vi "Apply styles to GObject.vi"(8 "Error in":errorcluster, 10 "Style Sheet":T1[](array[typedef]), 11 "Gen Refnum":refnum<vi>) -> (0 "Error out":errorcluster)   [LabVIEW 2019, in "LSS.lvlib"]
doc: "This VI takes the cluster of information from a pre-parsed style sheet and applies it to a front panel element. This VI will find which class/property needs to be set, cast the front panel generic element to the right class, then apply the property desired.\n\n<b>Inputs:</b>\n<b>Gen Refnum</b> - Reference to the front panel element which will be modified.\n<b>Style Sheet</b> - Pre-parsed style sheet containing only relevent properties to apply to the control specified by Gen Refnum.\n<b>Error In</b> - Standard Error In terminal.\n\n<b>Outputs</b>\n<b>Error Out</b> - Standard Error Out terminal."
uses:
  LSS.lvlib
  Controls/Style.ctl
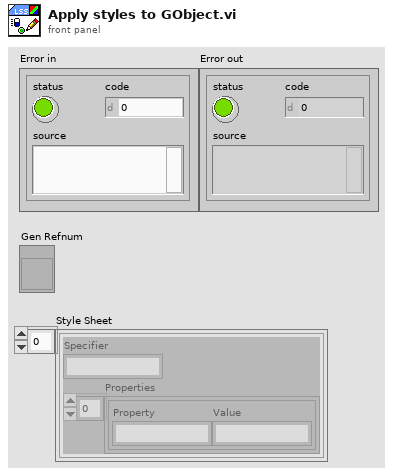
[diagram p1: front panel]
types:
  T1 = typedef "LSS.lvlib/Style.ctl" = cluster{"Specifier":string, "Properties":cluster{"Property":string, "Value":string}[]}
  T2 = enum8{"Enabled", "Disabled", "Disabled and Grayed Out"}
  T3 = enum16{"Always On", "Always Off", "Off While Running"}
  T4 = typedef "LVBoundsTypeDef.ctl" = cluster{"Width":u32, "Height":u32}
  T5 = typedef "LVRectTypeDef.ctl" = cluster{"Left":i16, "Top":i16, "Right":i16, "Bottom":i16}
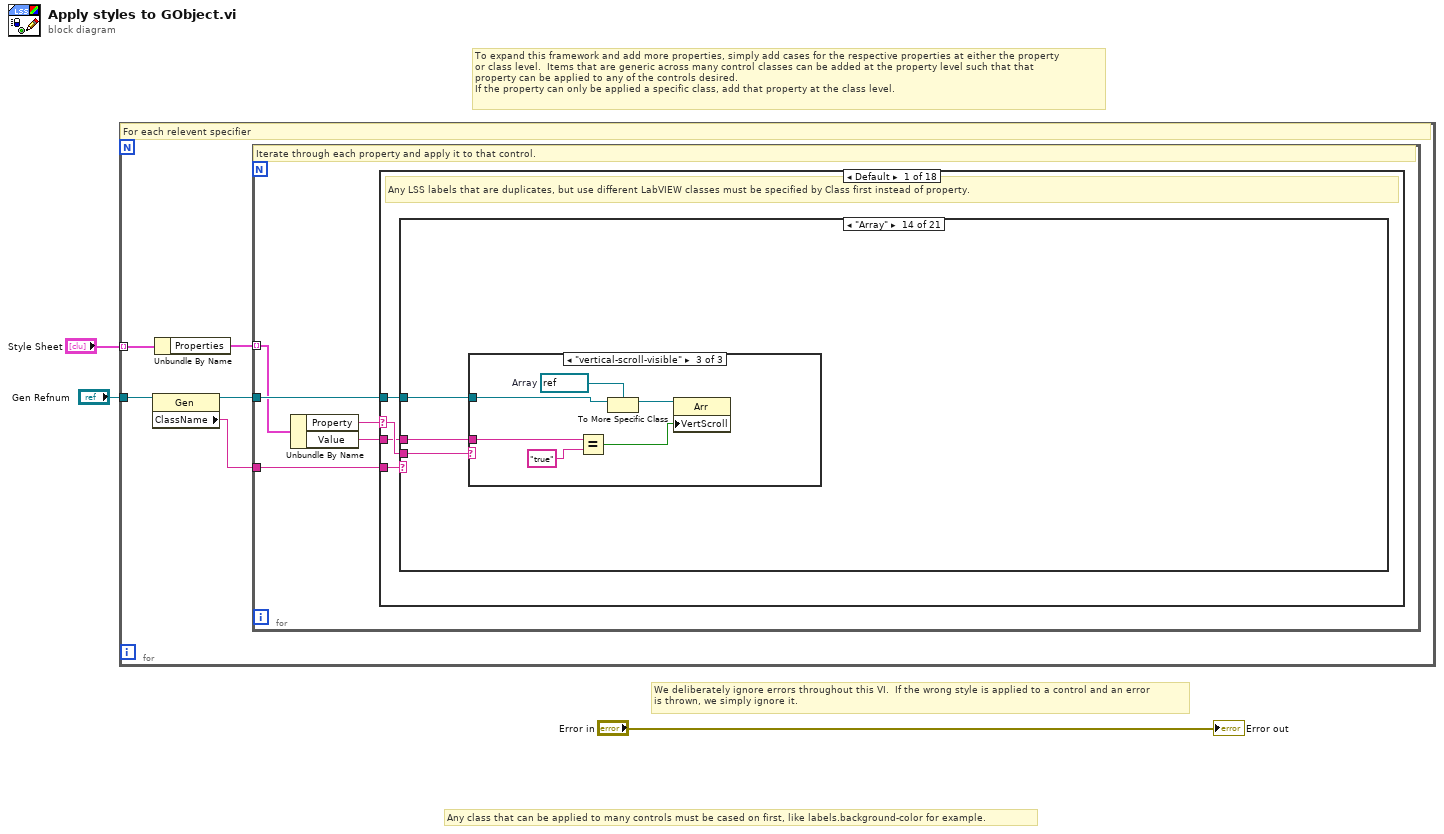
[diagram p0: block diagram]
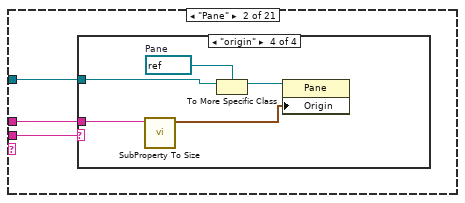
[diagram p3: hidden frame]
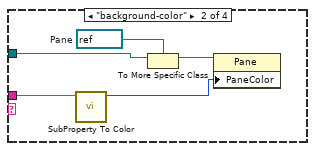
[diagram p5: hidden frame]
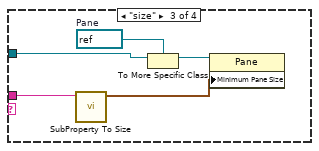
[diagram p6: hidden frame]
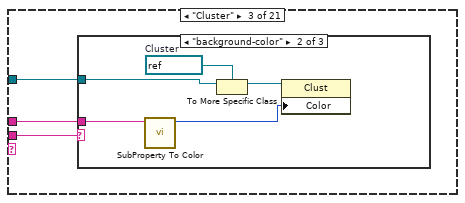
[diagram p7: hidden frame]
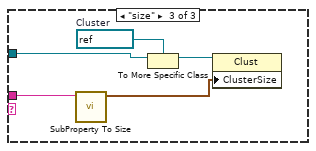
[diagram p9: hidden frame]
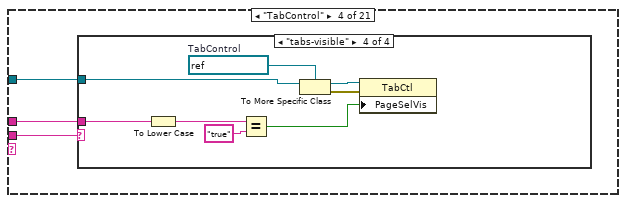
[diagram p10: hidden frame]
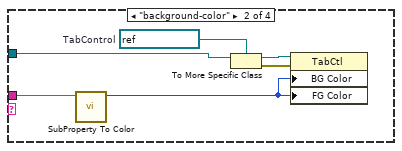
[diagram p12: hidden frame]
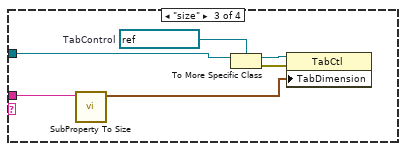
[diagram p13: hidden frame]
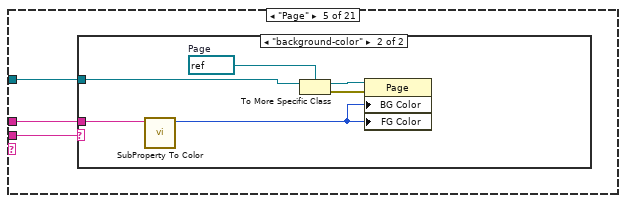
[diagram p14: hidden frame]
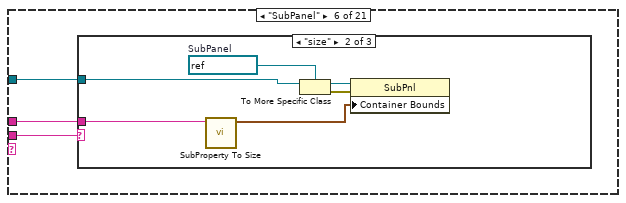
[diagram p16: hidden frame]
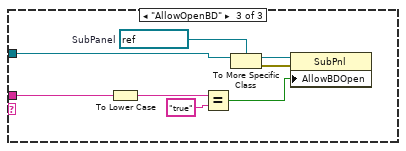
[diagram p18: hidden frame]
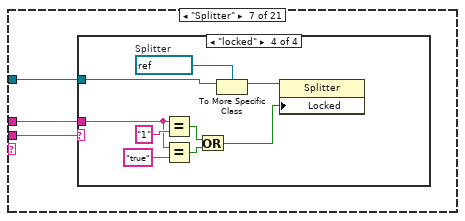
[diagram p19: hidden frame]
diagram:
  # "To expand this framework and add more properties, simply add cases for the respective properties at either the property\nor class level.  Items that are generic across many control classes can be added at the property level such that that \nproperty can be applied to any of the controls desired.\nIf the property can only be applied a specific class, add that property at the class level."
  # "Any class that can be applied to many controls must be cased on first, like labels.background-color for example."
  # "We deliberately ignore errors throughout this VI.  If the wrong style is applied to a control and an error\nis thrown, we simply ignore it."
  n1 = for {
    tunnel: "Style Sheet" -> [w8] mode=indexing
    tunnel: "Gen Refnum" -> [w6]
    # "For each relevent specifier"
    n2 = property class="Gen"(reference=w6) -> (reference out=w4:refnum<vi>, "ClassName"=w5:string)  [unwired: 1 in, 1 out]
    n3 = Unbundle By Name(w8) -> ("Properties"=w7:cluster{"Property":string, "Value":string}[])
    n4 = for {
      tunnel: w4 -> [w12]
      tunnel: w5 -> [w10]
      tunnel: w7 -> [w9] mode=indexing
      # "Iterate through each property and apply it to that control."
      n5 = Unbundle By Name(w9) -> ("Property"=w13:string, "Value"=w11:string)
      n6 = case shown="Default" w13 {
        selector: w13 -> [w16 _ _ _ _ _ _ _ _ _ _ _ _ _ _ _ _ _]
        tunnel: w12 -> [w15 w453 w458 w464 w470 w477 w483 w489 w494 w500 w507 w518 w524 w541 w555 w565 w575 w576]
        tunnel: w11 -> [w14 w449 w454 w459 w465 w473 w479 w484 w490 w495 w503 w517 w519 w530 w544 w561 w571 w579]
        tunnel: w10 -> [w17 _ _ _ _ _ _ _ _ _ _ _ _ _ _ _ _ _]
        frame Default {
          # "Any LSS labels that are duplicates, but use different LabVIEW classes must be specified by Class first instead of property."
          n7 = case shown="\"Array\"" w17 {
            selector: w17 -> [_ _ _ _ _ _ _ _ _ _ _ _ _ _ _ w255 _ _ _ _ _]
            tunnel: w16 -> [_ w20 w38 w51 w74 w83 w100 w122 w135 w153 w161 w174 w198 w220 w234 w258 w297 w324 w357 w436 w444]
            tunnel: w15 -> [_ w19 w37 w50 w73 w82 w99 w121 w134 w152 w160 w172 w197 w219 w233 w257 w296 w323 w355 w435 w443]
            tunnel: w14 -> [_ w18 w36 w49 w72 w81 w98 w120 w133 w151 w159 w173 w196 w218 w232 w256 w295 w322 w356 w432 w440]
            frame Default {
            }
            frame "Pane" {
              n8 = case shown="\"origin\"" w20 {
                tunnel: w19 -> [_ w25 w30 w35]
                tunnel: w18 -> [_ w22 w27 w32]
                frame Default {
                }
                frame "background-color" {
                  w24 = refnum<vi> refnum  # Pane
                  n9 = call "SubProperty To Color.vi"("Value"=w22) -> ("Color"=w21:u32)  [unwired: 10 in]
                  n10 = To More Specific Class(target class=w24, reference=w25) -> (specific class reference=w23:refnum<vi>)  [unwired: 1 in, 1 out]
                  n11 = property class="Pane"(reference=w23, "PaneColor"=w21) -> ()  [unwired: 1 in, 2 out]
                }
                frame "size" {
                  w29 = refnum<vi> refnum  # Pane
                  n12 = call "SubProperty To Size.vi"("SubProperty"=w27) -> ("Size"=w26:T4)  [unwired: 10 in]
                  n13 = To More Specific Class(target class=w29, reference=w30) -> (specific class reference=w28:refnum<vi>)  [unwired: 1 in, 1 out]
                  n14 = property class="Pane"(reference=w28, "Minimum Pane Size"=w26) -> ()  [unwired: 1 in, 2 out]
                }
                frame "origin" {
                  w34 = refnum<vi> refnum  # Pane
                  n15 = call "SubProperty To Size.vi"("SubProperty"=w32) -> ("Size"=w31:T4)  [unwired: 10 in]
                  n16 = To More Specific Class(target class=w34, reference=w35) -> (specific class reference=w33:refnum<vi>)  [unwired: 1 in, 1 out]
                  n17 = property class="Pane"(reference=w33, "Origin"=w31) -> ()  [unwired: 1 in, 2 out]
                }
              }
            }
            frame "Cluster" {
              n18 = case shown="\"background-color\"" w38 {
                tunnel: w37 -> [_ w43 w48]
                tunnel: w36 -> [_ w40 w45]
                frame Default {
                }
                frame "background-color" {
                  w42 = refnum<vi> refnum  # Cluster
                  n19 = call "SubProperty To Color.vi"("Value"=w40) -> ("Color"=w39:u32)  [unwired: 10 in]
                  n20 = To More Specific Class(target class=w42, reference=w43) -> (specific class reference=w41:refnum<vi>)  [unwired: 1 in, 1 out]
                  n21 = property class="Clust"(reference=w41, "Color"=w39) -> ()  [unwired: 1 in, 2 out]
                }
                frame "size" {
                  w47 = refnum<vi> refnum  # Cluster
                  n22 = call "SubProperty To Size.vi"("SubProperty"=w45) -> ("Size"=w44:T4)  [unwired: 10 in]
                  n23 = To More Specific Class(target class=w47, reference=w48) -> (specific class reference=w46:refnum<vi>)  [unwired: 1 in, 1 out]
                  n24 = property class="Clust"(reference=w46, "ClusterSize"=w44) -> ()  [unwired: 1 in, 2 out]
                }
              }
            }
            frame "TabControl" {
              n25 = case shown="\"tabs-visible\"" w51 {
                tunnel: w50 -> [_ w57 w63 w71]
                tunnel: w49 -> [_ w54 w60 w64]
                frame Default {
                }
                frame "background-color" {
                  w56 = refnum<vi> refnum  # TabControl
                  n26 = call "SubProperty To Color.vi"("Value"=w54) -> ("Color"=w52:u32)  [unwired: 10 in]
                  n27 = To More Specific Class(target class=w56, reference=w57) -> (specific class reference=w55:refnum<vi>, error out=w53:errorcluster)  [unwired: 1 in]
                  n28 = property class="TabCtl"(reference=w55, error in=w53, "BG Color"=w52, "FG Color"=w52) -> ()  [unwired: 2 out]
                }
                frame "size" {
                  w62 = refnum<vi> refnum  # TabControl
                  n29 = call "SubProperty To Size.vi"("SubProperty"=w60) -> ("Size"=w58:T4)  [unwired: 10 in]
                  n30 = To More Specific Class(target class=w62, reference=w63) -> (specific class reference=w61:refnum<vi>, error out=w59:errorcluster)  [unwired: 1 in]
                  n31 = property class="TabCtl"(reference=w61, error in=w59, "TabDimension"=w58) -> ()  [unwired: 2 out]
                }
                frame "tabs-visible" {
                  w70 = refnum<vi> refnum  # TabControl
                  n32 = To Lower Case(string=w64) -> (all lower case string=w66:string)
                  n33 = Equal?(x=w66, y="true") -> (x = y?=w65:bool)
                  n34 = To More Specific Class(target class=w70, reference=w71) -> (specific class reference=w69:refnum<vi>, error out=w68:errorcluster)  [unwired: 1 in]
                  n35 = property class="TabCtl"(reference=w69, error in=w68, "PageSelVis"=w65) -> ()  [unwired: 2 out]
                }
              }
            }
            frame "Page" {
              n36 = case shown="\"background-color\"" w74 {
                tunnel: w73 -> [_ w80]
                tunnel: w72 -> [_ w77]
                frame Default {
                }
                frame "background-color" {
                  w79 = refnum<vi> refnum  # Page
                  n37 = call "SubProperty To Color.vi"("Value"=w77) -> ("Color"=w75:u32)  [unwired: 10 in]
                  n38 = To More Specific Class(target class=w79, reference=w80) -> (specific class reference=w78:refnum<vi>, error out=w76:errorcluster)  [unwired: 1 in]
                  n39 = property class="Page"(reference=w78, error in=w76, "BG Color"=w75, "FG Color"=w75) -> ()  [unwired: 2 out]
                }
              }
            }
            frame "SubPanel" {
              n40 = case shown="\"size\"" w83 {
                tunnel: w82 -> [_ w89 w97]
                tunnel: w81 -> [_ w87 w91]
                frame Default {
                }
                frame "size" {
                  w88 = refnum<vi> refnum  # SubPanel
                  n41 = call "SubProperty To Size.vi"("SubProperty"=w87) -> ("Size"=w84:T4)  [unwired: 10 in]
                  n42 = To More Specific Class(target class=w88, reference=w89) -> (specific class reference=w86:refnum<vi>, error out=w85:errorcluster)  [unwired: 1 in]
                  n43 = property on="Property Node" class="SubPnl"(reference=w86, error in=w85, "Container Bounds"=w84) -> ()  [unwired: 2 out]
                }
                frame "AllowOpenBD" {
                  w96 = refnum<vi> refnum  # SubPanel
                  n44 = To Lower Case(string=w91) -> (all lower case string=w92:string)
                  n45 = Equal?(x=w92, y="true") -> (x = y?=w90:bool)
                  n46 = To More Specific Class(target class=w96, reference=w97) -> (specific class reference=w95:refnum<vi>, error out=w94:errorcluster)  [unwired: 1 in]
                  n47 = property on="Property Node" class="SubPnl"(reference=w95, error in=w94, "AllowBDOpen"=w90) -> ()  [unwired: 2 out]
                }
              }
            }
            frame "Splitter" {
              n48 = case shown="\"locked\"" w100 {
                tunnel: w99 -> [_ w105 w110 w119]
                tunnel: w98 -> [_ w102 w107 w113]
                frame Default {
                }
                frame "background-color" {
                  w104 = refnum<vi> refnum  # Splitter
                  n49 = call "SubProperty To Color.vi"("Value"=w102) -> ("Color"=w101:u32)  [unwired: 10 in]
                  n50 = To More Specific Class(target class=w104, reference=w105) -> (specific class reference=w103:refnum<vi>)  [unwired: 1 in, 1 out]
                  n51 = property class="Splitter"(reference=w103, "FGColor"=w101, "BGColor"=w101) -> ()  [unwired: 1 in, 2 out]
                }
                frame "splitter-position" {
                  w109 = refnum<vi> refnum  # Splitter
                  n52 = Decimal String To Number(string=w107) -> (number=w106:i32)  [unwired: 2 in, 1 out]
                  n53 = To More Specific Class(target class=w109, reference=w110) -> (specific class reference=w108:refnum<vi>)  [unwired: 1 in, 1 out]
                  n54 = property class="Splitter"(reference=w108, "Position"=w106) -> ()  [unwired: 1 in, 2 out]
                }
                frame "locked" {
                  w118 = refnum<vi> refnum  # Splitter
                  n55 = Equal?(x=w113, y="1") -> (x = y?=w116:bool)
                  n56 = Equal?(x=w113, y="true") -> (x = y?=w112:bool)
                  n57 = Or(x=w116, y=w112) -> (x .or. y?=w111:bool)
                  n58 = To More Specific Class(target class=w118, reference=w119) -> (specific class reference=w117:refnum<vi>)  [unwired: 1 in, 1 out]
                  n59 = property class="Splitter"(reference=w117, "Locked"=w111) -> ()  [unwired: 1 in, 2 out]
                }
              }
            }
            frame "RadioButtonsControl" {
              n60 = case shown="\"background-color\"" w122 {
                tunnel: w121 -> [_ w127 w132]
                tunnel: w120 -> [_ w124 w129]
                frame Default {
                }
                frame "background-color" {
                  w126 = refnum<vi> refnum  # RadioButtonsControl
                  n61 = call "SubProperty To Color.vi"("Value"=w124) -> ("Color"=w123:u32)  [unwired: 10 in]
                  n62 = To More Specific Class(target class=w126, reference=w127) -> (specific class reference=w125:refnum<vi>)  [unwired: 1 in, 1 out]
                  n63 = property class="RadioBtnsControl"(reference=w125, "Color"=w123) -> ()  [unwired: 1 in, 2 out]
                }
                frame "size" {
                  w131 = refnum<vi> refnum  # RadioButtonsControl
                  n64 = call "SubProperty To Size.vi"("SubProperty"=w129) -> ("Size"=w128:T4)  [unwired: 10 in]
                  n65 = To More Specific Class(target class=w131, reference=w132) -> (specific class reference=w130:refnum<vi>)  [unwired: 1 in, 1 out]
                  n66 = property class="RadioBtnsControl"(reference=w130, "ClusterSize"=w128) -> ()  [unwired: 1 in, 2 out]
                }
              }
            }
            frame "Decoration" {
              n67 = case shown="\"width\"" w135 {
                tunnel: w134 -> [_ w140 w145 w150]
                tunnel: w133 -> [_ w137 w142 w147]
                frame Default {
                }
                frame "background-color" {
                  w139 = refnum<vi> refnum  # Decoration
                  n68 = call "SubProperty To Color.vi"("Value"=w137) -> ("Color"=w136:u32)  [unwired: 10 in]
                  n69 = To More Specific Class(target class=w139, reference=w140) -> (specific class reference=w138:refnum<vi>)  [unwired: 1 in, 1 out]
                  n70 = property class="Decor"(reference=w138, "BG Color"=w136, "FG Color"=w136) -> ()  [unwired: 1 in, 2 out]
                }
                frame "size" {
                  w144 = refnum<vi> refnum  # Decoration
                  n71 = call "SubProperty To Size.vi"("SubProperty"=w142) -> ("Size"=w141:T4)  [unwired: 10 in]
                  n72 = To More Specific Class(target class=w144, reference=w145) -> (specific class reference=w143:refnum<vi>)  [unwired: 1 in, 1 out]
                  n73 = property class="Decor"(reference=w143, "Size"=w141) -> ()  [unwired: 1 in, 2 out]
                }
                frame "width" {
                  w149 = refnum<vi> refnum  # Decoration
                  n74 = Decimal String To Number(string=w147) -> (number=w146:i32)  [unwired: 2 in, 1 out]
                  n75 = To More Specific Class(target class=w149, reference=w150) -> (specific class reference=w148:refnum<vi>)  [unwired: 1 in, 1 out]
                  n76 = property class="Decor"(reference=w148, "Width"=w146) -> ()  [unwired: 1 in, 2 out]
                }
              }
            }
            frame "ActiveXContainer" {
              n77 = case shown="\"size\"" w153 {
                tunnel: w152 -> [_ w158]
                tunnel: w151 -> [_ w155]
                frame Default {
                }
                frame "size" {
                  w157 = refnum<vi> refnum  # ActiveXContainer
                  n78 = call "SubProperty To Size.vi"("SubProperty"=w155) -> ("Size"=w154:T4)  [unwired: 10 in]
                  n79 = To More Specific Class(target class=w157, reference=w158) -> (specific class reference=w156:refnum<vi>)  [unwired: 1 in, 1 out]
                  n80 = property class="AXCont"(reference=w156, "Container Bounds"=w154) -> ()  [unwired: 1 in, 2 out]
                }
              }
            }
            frame "Picture" {
              n81 = case shown="\"size\"" w161 {
                tunnel: w160 -> [_ w166 w171]
                tunnel: w159 -> [_ w163 w168]
                frame Default {
                }
                frame "size" {
                  w165 = refnum<vi> refnum  # Picture
                  n82 = call "SubProperty To Size.vi"("SubProperty"=w163) -> ("Size"=w162:T4)  [unwired: 10 in]
                  n83 = To More Specific Class(target class=w165, reference=w166) -> (specific class reference=w164:refnum<vi>)  [unwired: 1 in, 1 out]
                  n84 = property class="Pict"(reference=w164, "Draw Area Size"=w162) -> ()  [unwired: 1 in, 2 out]
                }
                frame "zoom" {
                  w170 = refnum<vi> refnum  # Picture
                  n85 = Fract/Exp String To Number(string=w168) -> (number=w167:dbl)  [unwired: 3 in, 1 out]
                  n86 = To More Specific Class(target class=w170, reference=w171) -> (specific class reference=w169:refnum<vi>)  [unwired: 1 in, 1 out]
                  n87 = property class="Pict"(reference=w169, "ZoomFactor"=w167) -> ()  [unwired: 1 in, 2 out]
                }
              }
            }
            frame "Boolean" {
              n88 = case shown="\"size\"" w174 {
                selector: w174 -> [w175 _ _ _ _]
                tunnel: w172 -> [_ w181 w186 w191 w195]
                tunnel: w173 -> [_ w178 w183 w188 w192]
                tunnel: [w175 _ _ _ _] -> _
                tunnel: [_ w176 _ _ _] -> _
                frame Default {
                }
                frame "size" {
                  w180 = refnum<vi> refnum  # Boolean
                  n89 = call "SubProperty To Size.vi"("SubProperty"=w178) -> ("Size"=w177:T4)  [unwired: 10 in]
                  n90 = To More Specific Class(target class=w180, reference=w181) -> (specific class reference=w179:refnum<vi>)  [unwired: 1 in, 1 out]
                  n91 = property class="Bool"(reference=w179, "Button Size"=w177) -> (error out=w176:errorcluster)  [unwired: 1 in, 1 out]
                }
                frame "font-size" {
                  w185 = refnum<vi> refnum  # Boolean
                  n92 = Decimal String To Number(string=w183) -> (number=w182:i32)  [unwired: 2 in, 1 out]
                  n93 = To More Specific Class(target class=w185, reference=w186) -> (specific class reference=w184:refnum<vi>)  [unwired: 1 in, 1 out]
                  n94 = property class="Bool"(reference=w184, "BoolText.FontSize"=w182) -> ()  [unwired: 1 in, 2 out]
                }
                frame "font-color" {
                  w190 = refnum<vi> refnum  # Boolean
                  n95 = call "SubProperty To Color.vi"("Value"=w188) -> ("Color"=w187:u32)  [unwired: 10 in]
                  n96 = To More Specific Class(target class=w190, reference=w191) -> (specific class reference=w189:refnum<vi>)  [unwired: 1 in, 1 out]
                  n97 = property class="Bool"(reference=w189, "BoolText.FontColor"=w187) -> ()  [unwired: 1 in, 2 out]
                }
                frame "font-name" {
                  w194 = refnum<vi> refnum  # Boolean
                  n98 = To More Specific Class(target class=w194, reference=w195) -> (specific class reference=w193:refnum<vi>)  [unwired: 1 in, 1 out]
                  n99 = property class="Bool"(reference=w193, "BoolText.FontName"=w192) -> ()  [unwired: 1 in, 2 out]
                }
              }
            }
            frame "Text" {
              n100 = case shown="\"background-color\"" w198 {
                tunnel: w197 -> [_ w203 w208 w213 w217]
                tunnel: w196 -> [_ w200 w205 w210 w214]
                frame Default {
                }
                frame "background-color" {
                  w202 = refnum<vi> refnum  # Text
                  n101 = call "SubProperty To Color.vi"("Value"=w200) -> ("Color"=w199:u32)  [unwired: 10 in]
                  n102 = To More Specific Class(target class=w202, reference=w203) -> (specific class reference=w201:refnum<vi>)  [unwired: 1 in, 1 out]
                  n103 = property class="Txt"(reference=w201, "BGColor"=w199, "FG Color"=w199) -> ()  [unwired: 1 in, 2 out]
                }
                frame "font-color" {
                  w207 = refnum<vi> refnum  # Text
                  n104 = call "SubProperty To Color.vi"("Value"=w205) -> ("Color"=w204:u32)  [unwired: 10 in]
                  n105 = To More Specific Class(target class=w207, reference=w208) -> (specific class reference=w206:refnum<vi>)  [unwired: 1 in, 1 out]
                  n106 = property class="Txt"(reference=w206, "TextColor"=w204) -> ()  [unwired: 1 in, 2 out]
                }
                frame "font-size" {
                  w212 = refnum<vi> refnum  # Text
                  n107 = Decimal String To Number(string=w210) -> (number=w209:i32)  [unwired: 2 in, 1 out]
                  n108 = To More Specific Class(target class=w212, reference=w213) -> (specific class reference=w211:refnum<vi>)  [unwired: 1 in, 1 out]
                  n109 = property class="Txt"(reference=w211, "FontSize"=w209) -> ()  [unwired: 1 in, 2 out]
                }
                frame "font-name" {
                  w216 = refnum<vi> refnum  # Text
                  n110 = To More Specific Class(target class=w216, reference=w217) -> (specific class reference=w215:refnum<vi>)  [unwired: 1 in, 1 out]
                  n111 = property class="Txt"(reference=w215, "FontName"=w214) -> ()  [unwired: 1 in, 2 out]
                }
              }
            }
            frame "Array" {
              n112 = case shown="\"vertical-scroll-visible\"" w220 {
                tunnel: w219 -> [_ w225 w231]
                tunnel: w218 -> [_ w222 w227]
                frame Default {
                }
                frame "numRows" {
                  w224 = refnum<vi> refnum  # Array
                  n113 = Decimal String To Number(string=w222) -> (number=w221:i32)  [unwired: 2 in, 1 out]
                  n114 = To More Specific Class(target class=w224, reference=w225) -> (specific class reference=w223:refnum<vi>)  [unwired: 1 in, 1 out]
                  n115 = property class="Arr"(reference=w223, "Number of Rows"=w221) -> ()  [unwired: 1 in, 2 out]
                }
                frame "vertical-scroll-visible" {
                  w230 = refnum<vi> refnum  # Array
                  n116 = Equal?(x=w227, y="true") -> (x = y?=w226:bool)
                  n117 = To More Specific Class(target class=w230, reference=w231) -> (specific class reference=w229:refnum<vi>)  [unwired: 1 in, 1 out]
                  n118 = property class="Arr"(reference=w229, "VertScroll"=w226) -> ()  [unwired: 1 in, 2 out]
                }
              }
            }
            frame "Enum", "Ring" {
              n119 = case shown="\"background-color\"" w234 {
                tunnel: w233 -> [_ w240 w245 w250 w254]
                tunnel: w232 -> [_ w238 w243 w248 w251]
                tunnel: [_ w235 _ _ _] -> _
                frame Default {
                }
                frame "background-color" {
                  w239 = refnum<vi> refnum  # NamedNumeric
                  n120 = call "SubProperty To Color.vi"("Value"=w238) -> ("Color"=w236:u32)  [unwired: 10 in]
                  n121 = To More Specific Class(target class=w239, reference=w240) -> (specific class reference=w237:refnum<vi>)  [unwired: 1 in, 1 out]
                  n122 = property on="Property Node" class="NmdNum"(reference=w237, "RingText.BG Color"=w236, "RingText.BGColor"=w236) -> (error out=w235:errorcluster)  [unwired: 1 in, 1 out]
                }
                frame "font-color" {
                  w241 = refnum<vi> refnum  # NamedNumeric
                  n123 = call "SubProperty To Color.vi"("Value"=w243) -> ("Color"=w242:u32)  [unwired: 10 in]
                  n124 = To More Specific Class(target class=w241, reference=w245) -> (specific class reference=w244:refnum<vi>)  [unwired: 1 in, 1 out]
                  n125 = property class="NmdNum"(reference=w244, "RingText.TextColor"=w242) -> ()  [unwired: 1 in, 2 out]
                }
                frame "font-size" {
                  w247 = refnum<vi> refnum  # NamedNumeric
                  n126 = Decimal String To Number(string=w248) -> (number=w246:i32)  [unwired: 2 in, 1 out]
                  n127 = To More Specific Class(target class=w247, reference=w250) -> (specific class reference=w249:refnum<vi>)  [unwired: 1 in, 1 out]
                  n128 = property class="NmdNum"(reference=w249, "RingText.FontSize"=w246) -> ()  [unwired: 1 in, 2 out]
                }
                frame "font-name" {
                  w252 = refnum<vi> refnum  # NamedNumeric
                  n129 = To More Specific Class(target class=w252, reference=w254) -> (specific class reference=w253:refnum<vi>)  [unwired: 1 in, 1 out]
                  n130 = property class="NmdNum"(reference=w253, "RingText.FontName"=w251) -> ()  [unwired: 1 in, 2 out]
                }
              }
            }
            frame "Knob", "Slide" {
              n131 = case shown="\"color\"" w258 {
                tunnel: w257 -> [_ w263 w266 w281 w284]
                tunnel: w256 -> [_ w260 w265 w278 w283]
                tunnel: w255 -> [_ _ w264 _ w282]
                frame Default {
                }
                frame "background-color" {
                  w262 = refnum<vi> refnum  # NumericWithScale
                  n132 = call "SubProperty To Color.vi"("Value"=w260) -> ("Color"=w259:u32)  [unwired: 10 in]
                  n133 = To More Specific Class(target class=w262, reference=w263) -> (specific class reference=w261:refnum<vi>)  [unwired: 1 in, 1 out]
                  n134 = property class="NumWthScl"(reference=w261, "BGColor"=w259, "FGColor"=w259) -> ()  [unwired: 1 in, 2 out]
                }
                frame "color" {
                  n135 = case shown="\"Slide\"" w264 {
                    tunnel: w266 -> [w271 w276]
                    tunnel: w265 -> [w268 w273]
                    frame "Slide" {
                      w270 = refnum<vi> refnum  # Slide
                      n136 = call "SubProperty To Color.vi"("Value"=w268) -> ("Color"=w267:u32)  [unwired: 10 in]
                      n137 = To More Specific Class(target class=w270, reference=w271) -> (specific class reference=w269:refnum<vi>)  [unwired: 1 in, 1 out]
                      n138 = property class="Slide"(reference=w269, "Fill Color"=w267) -> ()  [unwired: 1 in, 2 out]
                    }
                    frame "Knob", Default {
                      w275 = refnum<vi> refnum  # Knob
                      n139 = call "SubProperty To Color.vi"("Value"=w273) -> ("Color"=w272:u32)  [unwired: 10 in]
                      n140 = To More Specific Class(target class=w275, reference=w276) -> (specific class reference=w274:refnum<vi>)  [unwired: 1 in, 1 out]
                      n141 = property class="Knob"(reference=w274, "BG Color"=w272, "FG Color"=w272) -> ()  [unwired: 1 in, 2 out]
                    }
                  }
                }
                frame "size" {
                  w280 = refnum<vi> refnum  # NumericWithScale
                  n142 = call "SubProperty To Size.vi"("SubProperty"=w278) -> ("Size"=w277:T4)  [unwired: 10 in]
                  n143 = To More Specific Class(target class=w280, reference=w281) -> (specific class reference=w279:refnum<vi>)  [unwired: 1 in, 1 out]
                  n144 = property class="NumWthScl"(reference=w279, "Housing Size"=w277) -> ()  [unwired: 1 in, 2 out]
                }
                frame "font-color" {
                  n145 = case shown="\"Slide\"" w282 {
                    tunnel: w284 -> [w287 w294]
                    tunnel: w283 -> [w286 w291]
                    frame "Knob", Default {
                      w289 = refnum<vi> refnum  # Knob
                      n146 = call "SubProperty To Color.vi"("Value"=w286) -> ("Color"=w285:u32)  [unwired: 10 in]
                      n147 = To More Specific Class(target class=w289, reference=w287) -> (specific class reference=w288:refnum<vi>)  [unwired: 1 in, 1 out]
                      n148 = property class="Knob"(reference=w288, "Scale.Marker.TextColor"=w285, "Scale.MinorTickColor"=w285, "Scale.TickColor"=w285) -> ()  [unwired: 1 in, 2 out]
                    }
                    frame "Slide" {
                      w293 = refnum<vi> refnum  # Slide
                      n149 = call "SubProperty To Color.vi"("Value"=w291) -> ("Color"=w290:u32)  [unwired: 10 in]
                      n150 = To More Specific Class(target class=w293, reference=w294) -> (specific class reference=w292:refnum<vi>)  [unwired: 1 in, 1 out]
                      n151 = property class="Slide"(reference=w292, "Scale.Marker.TextColor"=w290, "Scale.MinorTickColor"=w290, "Scale.TickColor"=w290) -> ()  [unwired: 1 in, 2 out]
                    }
                  }
                }
              }
            }
            frame "String" {
              n152 = case shown="\"size\"" w297 {
                tunnel: w296 -> [_ w302 w307 w312 w317 w321]
                tunnel: w295 -> [_ w299 w304 w309 w314 w318]
                frame Default {
                }
                frame "background-color" {
                  w301 = refnum<vi> refnum  # String
                  n153 = call "SubProperty To Color.vi"("Value"=w299) -> ("Color"=w298:u32)  [unwired: 10 in]
                  n154 = To More Specific Class(target class=w301, reference=w302) -> (specific class reference=w300:refnum<vi>)  [unwired: 1 in, 1 out]
                  n155 = property class="Str"(reference=w300, "Text.BGColor"=w298) -> ()  [unwired: 1 in, 2 out]
                }
                frame "font-color" {
                  w306 = refnum<vi> refnum  # String
                  n156 = call "SubProperty To Color.vi"("Value"=w304) -> ("Color"=w303:u32)  [unwired: 10 in]
                  n157 = To More Specific Class(target class=w306, reference=w307) -> (specific class reference=w305:refnum<vi>)  [unwired: 1 in, 1 out]
                  n158 = property class="Str"(reference=w305, "Text.TextColor"=w303) -> ()  [unwired: 1 in, 2 out]
                }
                frame "size" {
                  w311 = refnum<vi> refnum  # String
                  n159 = call "SubProperty To Size.vi"("SubProperty"=w309) -> ("Size"=w308:T4)  [unwired: 10 in]
                  n160 = To More Specific Class(target class=w311, reference=w312) -> (specific class reference=w310:refnum<vi>)  [unwired: 1 in, 1 out]
                  n161 = property class="Str"(reference=w310, "Size"=w308) -> ()  [unwired: 1 in, 2 out]
                }
                frame "font-size" {
                  w316 = refnum<vi> refnum  # String
                  n162 = Decimal String To Number(string=w314) -> (number=w313:i32)  [unwired: 2 in, 1 out]
                  n163 = To More Specific Class(target class=w316, reference=w317) -> (specific class reference=w315:refnum<vi>)  [unwired: 1 in, 1 out]
                  n164 = property class="Str"(reference=w315, "Text.FontSize"=w313) -> ()  [unwired: 1 in, 2 out]
                }
                frame "font-name" {
                  w320 = refnum<vi> refnum  # String
                  n165 = To More Specific Class(target class=w320, reference=w321) -> (specific class reference=w319:refnum<vi>)  [unwired: 1 in, 1 out]
                  n166 = property class="Str"(reference=w319, "Text.FontName"=w318) -> ()  [unwired: 1 in, 2 out]
                }
              }
            }
            frame "Digital" {
              n167 = case shown="\"background-color\"" w324 {
                tunnel: w323 -> [_ w329 w334 w340 w345 w349]
                tunnel: w322 -> [_ w326 w331 w337 w342 w346]
                frame Default {
                }
                frame "background-color" {
                  w328 = refnum<vi> refnum  # Digital
                  n168 = call "SubProperty To Color.vi"("Value"=w326) -> ("Color"=w325:u32)  [unwired: 10 in]
                  n169 = To More Specific Class(target class=w328, reference=w329) -> (specific class reference=w327:refnum<vi>)  [unwired: 1 in, 1 out]
                  n170 = property class="DigNum"(reference=w327, "NumText.BG Color"=w325, "NumText.FG Color"=w325, "NumText.BGColor"=w325) -> ()  [unwired: 1 in, 2 out]
                }
                frame "font-color" {
                  w333 = refnum<vi> refnum  # Digital
                  n171 = call "SubProperty To Color.vi"("Value"=w331) -> ("Color"=w330:u32)  [unwired: 10 in]
                  n172 = To More Specific Class(target class=w333, reference=w334) -> (specific class reference=w332:refnum<vi>)  [unwired: 1 in, 1 out]
                  n173 = property class="DigNum"(reference=w332, "NumText.TextColor"=w330) -> ()  [unwired: 1 in, 2 out]
                }
                frame "size" {
                  w339 = refnum<vi> refnum  # Digital
                  n174 = call "SubProperty To Size.vi"("SubProperty"=w337) -> ("Size"=w336:T4)  [unwired: 10 in]
                  n175 = Unbundle By Name(w336) -> ("Width"=w335:u32)
                  n176 = To More Specific Class(target class=w339, reference=w340) -> (specific class reference=w338:refnum<vi>)  [unwired: 1 in, 1 out]
                  n177 = property class="DigNum"(reference=w338, "Text Width"=w335) -> ()  [unwired: 1 in, 2 out]
                }
                frame "font-size" {
                  w344 = refnum<vi> refnum  # Digital
                  n178 = Decimal String To Number(string=w342) -> (number=w341:i32)  [unwired: 2 in, 1 out]
                  n179 = To More Specific Class(target class=w344, reference=w345) -> (specific class reference=w343:refnum<vi>)  [unwired: 1 in, 1 out]
                  n180 = property class="DigNum"(reference=w343, "NumText.FontSize"=w341) -> ()  [unwired: 1 in, 2 out]
                }
                frame "font-name" {
                  w348 = refnum<vi> refnum  # Digital
                  n181 = To More Specific Class(target class=w348, reference=w349) -> (specific class reference=w347:refnum<vi>)  [unwired: 1 in, 1 out]
                  n182 = property class="DigNum"(reference=w347, "NumText.FontName"=w346) -> ()  [unwired: 1 in, 2 out]
                }
              }
            }
            frame "DigitalGraph", "GraphChart", "WaveformChart", "WaveformGraph", "XYGraph" {
              w354 = refnum<vi> refnum  # GraphChart
              n183 = To More Specific Class(target class=w354, reference=w355) -> (specific class reference=w353:refnum<vi>, error out=w350:errorcluster)  [unwired: 1 in]
              n184 = case shown="\"size\"" w357 {
                tunnel: w356 -> [_ w370 w376 w382 w388 w394 w400 w402 w407 w417 w421 w425 w431]
                tunnel: w353 -> [w364 w367 w372 w378 w384 w390 w399 w406 w411 w413 w418 w422 w427]
                tunnel: [w364 w369 w374 w380 w386 w392 w397 w404 w409 w416 w418 w422 w430] -> w352
                tunnel: [w363 w368 w373 w379 w385 w391 w395 w403 w408 w415 w419 w423 w429] -> w351
                tunnel: w350 -> [w363 w366 w375 w381 w387 w393 w398 w405 w410 w414 w420 w424 w428]
                frame Default {
                }
                frame "graph.frame-color" {
                  n185 = call "SubProperty To Color.vi"("Value"=w370) -> ("Color"=w365:u32)  [unwired: 10 in]
                  n186 = property class="GrphChrt"(reference=w367, error in=w366, "XScale.UnitLabel.BGColor"=w365, "YScale.UnitLabel.BGColor"=w365, "XScale.NameLbl.BGColor"=w365, "YScale.NameLbl.BGColor"=w365, "XScale.Marker.BGColor"=w365, "YScale.Marker.BGColor"=w365) -> ()  [unwired: 2 out]
                  n187 = property class="GrphChrt"(reference=w367, error in=w366, "Frame Color"=w365) -> (reference out=w369:refnum<vi>, error out=w368:errorcluster)
                }
                frame "graph.grid-colors.major-x" {
                  n188 = call "SubProperty To Color.vi"("Value"=w376) -> ("Color"=w371:u32)  [unwired: 10 in]
                  n189 = property class="GrphChrt"(reference=w372, error in=w375, "XScale.MajGrdColor"=w371) -> (reference out=w374:refnum<vi>, error out=w373:errorcluster)
                }
                frame "graph.grid-colors.minor-x" {
                  n190 = call "SubProperty To Color.vi"("Value"=w382) -> ("Color"=w377:u32)  [unwired: 10 in]
                  n191 = property class="GrphChrt"(reference=w378, error in=w381, "XScale.MnrGrdColor"=w377) -> (reference out=w380:refnum<vi>, error out=w379:errorcluster)
                }
                frame "graph.grid-colors.major-y" {
                  n192 = call "SubProperty To Color.vi"("Value"=w388) -> ("Color"=w383:u32)  [unwired: 10 in]
                  n193 = property class="GrphChrt"(reference=w384, error in=w387, "YScale.MajGrdColor"=w383) -> (reference out=w386:refnum<vi>, error out=w385:errorcluster)
                }
                frame "graph.grid-colors.minor-y" {
                  n194 = call "SubProperty To Color.vi"("Value"=w394) -> ("Color"=w389:u32)  [unwired: 10 in]
                  n195 = property class="GrphChrt"(reference=w390, error in=w393, "YScale.MnrGrdColor"=w389) -> (reference out=w392:refnum<vi>, error out=w391:errorcluster)
                }
                frame "font-color" {
                  n196 = call "SubProperty To Color.vi"("Value"=w400) -> ("Color"=w396:u32)  [unwired: 10 in]
                  n197 = property class="GrphChrt"(reference=w399, error in=w398, "XScale.UnitLabel.TextColor"=w396, "YScale.UnitLabel.TextColor"=w396, "XScale.NameLbl.TextColor"=w396, "YScale.NameLbl.TextColor"=w396, "XScale.Marker.TextColor"=w396, "YScale.Marker.TextColor"=w396) -> (reference out=w397:refnum<vi>, error out=w395:errorcluster)
                }
                frame "font-size" {
                  n198 = Decimal String To Number(string=w402) -> (number=w401:i32)  [unwired: 2 in, 1 out]
                  n199 = property class="GrphChrt"(reference=w406, error in=w405, "XScale.UnitLabel.FontSize"=w401, "YScale.UnitLabel.FontSize"=w401, "XScale.NameLbl.FontSize"=w401, "YScale.NameLbl.FontSize"=w401, "XScale.Marker.FontSize"=w401, "YScale.Marker.FontSize"=w401) -> (reference out=w404:refnum<vi>, error out=w403:errorcluster)
                }
                frame "font-name" {
                  n200 = property class="GrphChrt"(reference=w411, error in=w410, "XScale.UnitLabel.FontName"=w407, "YScale.UnitLabel.FontName"=w407, "XScale.NameLbl.FontName"=w407, "YScale.NameLbl.FontName"=w407, "XScale.Marker.FontName"=w407, "YScale.Marker.FontName"=w407) -> (reference out=w409:refnum<vi>, error out=w408:errorcluster)
                }
                frame "background-color" {
                  n201 = call "SubProperty To Color.vi"("Value"=w417) -> ("Color"=w412:u32)  [unwired: 10 in]
                  n202 = property class="GrphChrt"(reference=w413, error in=w414, "BG Color"=w412) -> (reference out=w416:refnum<vi>, error out=w415:errorcluster)
                }
                frame "plot-color" {
                  n203 = call "Set Plot Color.vi"("error in (no error)"=w420, "Value"=w421, "GraphChart in"=w418) -> ("error out"=w419:errorcluster)  [unwired: 8 in]
                }
                frame "line-width" {
                  n204 = call "Set Line Width.vi"("error in (no error)"=w424, "Value"=w425, "GraphChart in"=w422) -> ("error out"=w423:errorcluster)  [unwired: 8 in]
                }
                frame "size" {
                  n205 = call "SubProperty To Size.vi"("SubProperty"=w431) -> ("Size"=w426:T4)  [unwired: 10 in]
                  n206 = property class="GrphChrt"(reference=w427, error in=w428, "Plot Area Size"=w426) -> (reference out=w430:refnum<vi>, error out=w429:errorcluster)
                }
              }
              n207 = case shown="No Error" w351 {
                selector: w351 -> [w359 _]
                tunnel: w352 -> [w360 _]
                frame No Error {
                  # "Do not delete this, it refreshes the \ngraph."
                  n208 = property on="Property Node" class="GrphChrt"(reference=w360, error in=w359) -> (reference out=w361:refnum<vi>, error out=w358:errorcluster, "Plot Bounds"=w362:T5)
                  n209 = property on="Property Node" class="GrphChrt"(reference=w361, error in=w358, "Plot Bounds"=w362) -> ()  [unwired: 2 out]
                }
                frame Error {
                }
              }
            }
            frame "Table" {
              w434 = refnum<vi> refnum  # Table
              n210 = To More Specific Class(target class=w434, reference=w435) -> (specific class reference=w433:refnum<vi>)  [unwired: 1 in, 1 out]
              n211 = case shown="\"size\"" w436 {
                tunnel: w433 -> [_ w439]
                tunnel: w432 -> [_ w438]
                frame Default {
                }
                frame "size" {
                  n212 = call "SubProperty To Size.vi"("SubProperty"=w438) -> ("Size"=w437:T4)  [unwired: 10 in]
                  n213 = property class="Tbl"(reference=w439, "Size"=w437) -> ()  [unwired: 1 in, 2 out]
                }
              }
            }
            frame "Listbox" {
              w442 = refnum<vi> refnum  # ListBox
              n214 = To More Specific Class(target class=w442, reference=w443) -> (specific class reference=w441:refnum<vi>)  [unwired: 1 in, 1 out]
              n215 = case shown="\"size\"" w444 {
                tunnel: w441 -> [_ w447]
                tunnel: w440 -> [_ w446]
                frame Default {
                }
                frame "size" {
                  n216 = call "SubProperty To Size.vi"("SubProperty"=w446) -> ("Size"=w445:T4)  [unwired: 10 in]
                  n217 = property class="LstBox"(reference=w447, "Size"=w445) -> ()  [unwired: 1 in, 2 out]
                }
              }
            }
          }
        }
        frame "labels.font-size" {
          w452 = refnum<vi> refnum  # Control
          n218 = Decimal String To Number(string=w449) -> (number=w448:i32)  [unwired: 2 in, 1 out]
          n219 = To More Specific Class(target class=w452, reference=w453) -> (specific class reference=w451:refnum<vi>, error out=w450:errorcluster)  [unwired: 1 in]
          n220 = property class="Ctl"(reference=w451, error in=w450, "Label.FontSize"=w448) -> ()  [unwired: 2 out]
        }
        frame "labels.font-name" {
          w457 = refnum<vi> refnum  # Control
          n221 = To More Specific Class(target class=w457, reference=w458) -> (specific class reference=w456:refnum<vi>, error out=w455:errorcluster)  [unwired: 1 in]
          n222 = property class="Ctl"(reference=w456, error in=w455, "Label.FontName"=w454) -> ()  [unwired: 2 out]
        }
        frame "labels.font-color" {
          w463 = refnum<vi> refnum  # Control
          n223 = call "SubProperty To Color.vi"("Value"=w459) -> ("Color"=w460:u32)  [unwired: 10 in]
          n224 = To More Specific Class(target class=w463, reference=w464) -> (specific class reference=w462:refnum<vi>, error out=w461:errorcluster)  [unwired: 1 in]
          n225 = property class="Ctl"(reference=w462, error in=w461, "Label.TextColor"=w460) -> ()  [unwired: 2 out]
        }
        frame "labels.background-color" {
          w469 = refnum<vi> refnum  # Control
          n226 = call "SubProperty To Color.vi"("Value"=w465) -> ("Color"=w466:u32)  [unwired: 10 in]
          n227 = To More Specific Class(target class=w469, reference=w470) -> (specific class reference=w468:refnum<vi>, error out=w467:errorcluster)  [unwired: 1 in]
          n228 = property class="Ctl"(reference=w468, error in=w467, "Label.BGColor"=w466) -> ()  [unwired: 2 out]
        }
        frame "labels.visible" {
          w476 = refnum<vi> refnum  # Control
          n229 = Equal?(x=w473, y="true") -> (x = y?=w471:bool)
          n230 = To More Specific Class(target class=w476, reference=w477) -> (specific class reference=w475:refnum<vi>, error out=w474:errorcluster)  [unwired: 1 in]
          n231 = property class="Ctl"(reference=w475, error in=w474, "Label.Visible"=w471) -> ()  [unwired: 2 out]
        }
        frame "captions.font-size" {
          w482 = refnum<vi> refnum  # Control
          n232 = Decimal String To Number(string=w479) -> (number=w478:i32)  [unwired: 2 in, 1 out]
          n233 = To More Specific Class(target class=w482, reference=w483) -> (specific class reference=w481:refnum<vi>, error out=w480:errorcluster)  [unwired: 1 in]
          n234 = property class="Ctl"(reference=w481, error in=w480, "Caption.FontSize"=w478) -> ()  [unwired: 2 out]
        }
        frame "captions.font-color" {
          w488 = refnum<vi> refnum  # Control
          n235 = call "SubProperty To Color.vi"("Value"=w484) -> ("Color"=w485:u32)  [unwired: 10 in]
          n236 = To More Specific Class(target class=w488, reference=w489) -> (specific class reference=w487:refnum<vi>, error out=w486:errorcluster)  [unwired: 1 in]
          n237 = property class="Ctl"(reference=w487, error in=w486, "Caption.TextColor"=w485) -> ()  [unwired: 2 out]
        }
        frame "captions.font-name" {
          w493 = refnum<vi> refnum  # Control
          n238 = To More Specific Class(target class=w493, reference=w494) -> (specific class reference=w492:refnum<vi>, error out=w491:errorcluster)  [unwired: 1 in]
          n239 = property class="Ctl"(reference=w492, error in=w491, "Caption.FontName"=w490) -> ()  [unwired: 2 out]
        }
        frame "captions.background-color" {
          w499 = refnum<vi> refnum  # Control
          n240 = call "SubProperty To Color.vi"("Value"=w495) -> ("Color"=w496:u32)  [unwired: 10 in]
          n241 = To More Specific Class(target class=w499, reference=w500) -> (specific class reference=w498:refnum<vi>, error out=w497:errorcluster)  [unwired: 1 in]
          n242 = property class="Ctl"(reference=w498, error in=w497, "Caption.BGColor"=w496) -> ()  [unwired: 2 out]
        }
        frame "captions.visible" {
          w506 = refnum<vi> refnum  # Control
          n243 = Equal?(x=w503, y="true") -> (x = y?=w501:bool)
          n244 = To More Specific Class(target class=w506, reference=w507) -> (specific class reference=w505:refnum<vi>, error out=w504:errorcluster)  [unwired: 1 in]
          n245 = property class="Ctl"(reference=w505, error in=w504, "Caption.Visible"=w501) -> ()  [unwired: 2 out]
        }
        frame "position" {
          w508 = refnum<vi> refnum  # GObject
          n246 = Match Pattern(string=w517, regular expression=",") -> (before substring=w515:string, after substring=w514:string)  [unwired: 1 in, 2 out]
          n247 = call <vilib>:"Trim Whitespace.vi"("string"=w515) -> ("trimmed string"=w511:string)  [unwired: 1 in]
          n248 = call <vilib>:"Trim Whitespace.vi"("string"=w514) -> ("trimmed string"=w513:string)  [unwired: 1 in]
          n249 = To More Specific Class(target class=w508, reference=w518) -> (specific class reference=w509:refnum<vi>)  [unwired: 1 in, 1 out]
          n250 = Decimal String To Number(string=w511) -> (number=w510:i32)  [unwired: 2 in, 1 out]
          n251 = Decimal String To Number(string=w513) -> (number=w512:i32)  [unwired: 2 in, 1 out]
          n252 = property class="GObj"(reference=w509, "Left"=w510, "Top"=w512) -> ()  [unwired: 1 in, 2 out]
        }
        frame "disabled-state" {
          w523 = refnum<vi> refnum  # Control
          n253 = case shown="\"disabled\", \"true\", Default" w519 {
            tunnel: [T2."Disabled" ("Disabled") T2."Disabled and Grayed Out" ("Disabled") T2."Enabled" ("Disabled")] -> w520
            frame "disabled", "true", Default {
            }
            frame "gray" {
            }
            frame "enabled", "false" {
            }
          }
          n254 = To More Specific Class(target class=w523, reference=w524) -> (specific class reference=w522:refnum<vi>, error out=w521:errorcluster)  [unwired: 1 in]
          n255 = property class="Ctl"(reference=w522, error in=w521, "DisabledEnum"=w520) -> ()  [unwired: 2 out]
        }
        frame "bool.true-color" {
          w540 = refnum<vi> refnum  # Boolean
          n256 = call "SubProperty To Color.vi"("Value"=w530) -> ("Color"=w534:u32)  [unwired: 10 in]
          n257 = To More Specific Class(target class=w540, reference=w541) -> (specific class reference=w538:refnum<vi>, error out=w539:errorcluster)  [unwired: 1 in]
          n258 = Bundle(cluster=cluster{u32, u32} {0, 0}, w534, w534) -> (w528:cluster{u32, u32})
          n259 = property class="Bool"(reference=w538, error in=w539) -> (reference out=w536:refnum<vi>, error out=w537:errorcluster, "Colors [4]"=w535:cluster{u32, u32}[])
          n260 = Replace Array Subset(array=w535, new element #1=w528, index #1=1 ("index"), new element #2=w528, index #2=3 ("index")) -> (w531:cluster{u32, u32}[])
          n261 = property class="Bool"(reference=w536, error in=w537, "Colors [4]"=w531) -> ()  [unwired: 2 out]
        }
        frame "bool.false-color" {
          w554 = refnum<vi> refnum  # Boolean
          n262 = call "SubProperty To Color.vi"("Value"=w544) -> ("Color"=w548:u32)  [unwired: 10 in]
          n263 = To More Specific Class(target class=w554, reference=w555) -> (specific class reference=w552:refnum<vi>, error out=w553:errorcluster)  [unwired: 1 in]
          n264 = Bundle(cluster=cluster{u32, u32} {0, 0}, w548, w548) -> (w542:cluster{u32, u32})
          n265 = property class="Bool"(reference=w552, error in=w553) -> (reference out=w550:refnum<vi>, error out=w551:errorcluster, "Colors [4]"=w549:cluster{u32, u32}[])
          n266 = Replace Array Subset(array=w549, new element #1=w542, index #1=0 ("index"), new element #2=w542, index #2=2 ("index")) -> (w545:cluster{u32, u32}[])
          n267 = property class="Bool"(reference=w550, error in=w551, "Colors [4]"=w545) -> ()  [unwired: 2 out]
        }
        frame "horizontal-scroll-bar" {
          w564 = refnum<vi> refnum  # Pane
          n268 = Equal?(x=w561, y="true") -> (x = y?=w559:bool)
          n269 = Select(t=T3."Always On" ("Horizontal Scrollbar Visibility"), s=w559, f=T3."Always Off" ("Horizontal Scrollbar Visibility")) -> (s? t:f=w556:T3)
          n270 = To More Specific Class(target class=w564, reference=w565) -> (specific class reference=w563:refnum<vi>, error out=w562:errorcluster)  [unwired: 1 in]
          n271 = property class="Pane"(reference=w563, error in=w562, "HorizScrollbarVisibility"=w556) -> ()  [unwired: 2 out]
        }
        frame "vertical-scroll-bar" {
          w574 = refnum<vi> refnum  # Pane
          n272 = Equal?(x=w571, y="true") -> (x = y?=w569:bool)
          n273 = Select(t=T3."Always On" ("Horizontal Scrollbar Visibility"), s=w569, f=T3."Always Off" ("Horizontal Scrollbar Visibility")) -> (s? t:f=w566:T3)
          n274 = To More Specific Class(target class=w574, reference=w575) -> (specific class reference=w573:refnum<vi>, error out=w572:errorcluster)  [unwired: 1 in]
          n275 = property class="Pane"(reference=w573, error in=w572, "VertScrollbarVisibility"=w566) -> ()  [unwired: 2 out]
        }
        frame "visible" {
          w582 = refnum<vi> refnum  # Control
          n276 = Equal?(x=w579, y="true") -> (x = y?=w577:bool)
          n277 = To More Specific Class(target class=w582, reference=w576) -> (specific class reference=w581:refnum<vi>, error out=w580:errorcluster)  [unwired: 1 in]
          n278 = case shown="Error" w580 {
            selector: w580 -> [w584 _]
            tunnel: w581 -> [w585 _]
            tunnel: w577 -> [w583 w587]
            tunnel: w576 -> [_ w589]
            frame No Error {
              n279 = property class="Ctl"(reference=w585, error in=w584, "Visible"=w583) -> ()  [unwired: 2 out]
            }
            frame Error {
              w590 = refnum<vi> refnum  # Decoration
              n280 = To More Specific Class(target class=w590, reference=w589) -> (specific class reference=w588:refnum<vi>, error out=w586:errorcluster)  [unwired: 1 in]
              n281 = property class="Decor"(reference=w588, error in=w586, "Visible"=w587) -> ()  [unwired: 2 out]
            }
          }
        }
      }
    }
  }
  "Error out" <- "Error in"
